vi "From Serial Form.vi"(6 "Serial Version":T1, 10 "Deserializer in":refnum<class "Deserializer.lvclass">, 11 "BrowerComponent in":refnum<class "BrowerComponent.lvclass">) -> (0 "error out":errorcluster, 2 "Deserializer out":refnum<class "Deserializer.lvclass">, 3 "BrowerComponent out":refnum<class "BrowerComponent.lvclass">)   [LabVIEW 2015, in "BrowerComponent.lvclass"]
uses:
  BrowerComponent.lvclass
  <vilib>/NI/AQ Character Lineator/Deserializer/Deserializer.lvclass
  <vilib>/NI/AQ Character Lineator/Serialization Common/Serial Version.ctl
  <vilib>/NI/AQ Character Lineator/Serializable/Remove String.vi
  <vilib>/NI/AQ Character Lineator/Serializable/Remove Int32.vi
  <vilib>/NI/AQ Character Lineator/Serializable Variant/Remove Variant.vi
  <vilib>/NI/AQ Character Lineator/Serializable/Serializable.lvclass
  <vilib>/NI/AQ Character Lineator/Serializable Variant/Serializable Variant.lvclass
  <vilib>/NI/AQ Character Lineator/Serialization Common/Serialization Common.lvlib
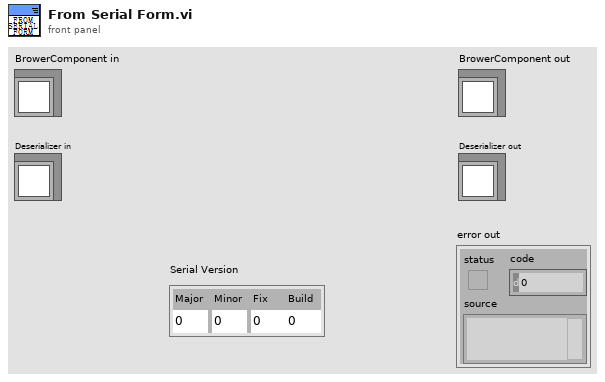
[diagram p1: front panel]
types:
  T1 = typedef "Serialization Common.lvlib/Serial Version.ctl" = cluster{"Major":u16, "Minor":u16, "Fix":u16, "Build":u16}
  T2 = typedef "BrowerComponent.lvclass/ObjectAttributes.ctl" = cluster{"ComponentID":string, "SymbolIndex":i32, "ComponentName":string, "PartsOfComponent_dict":variant}
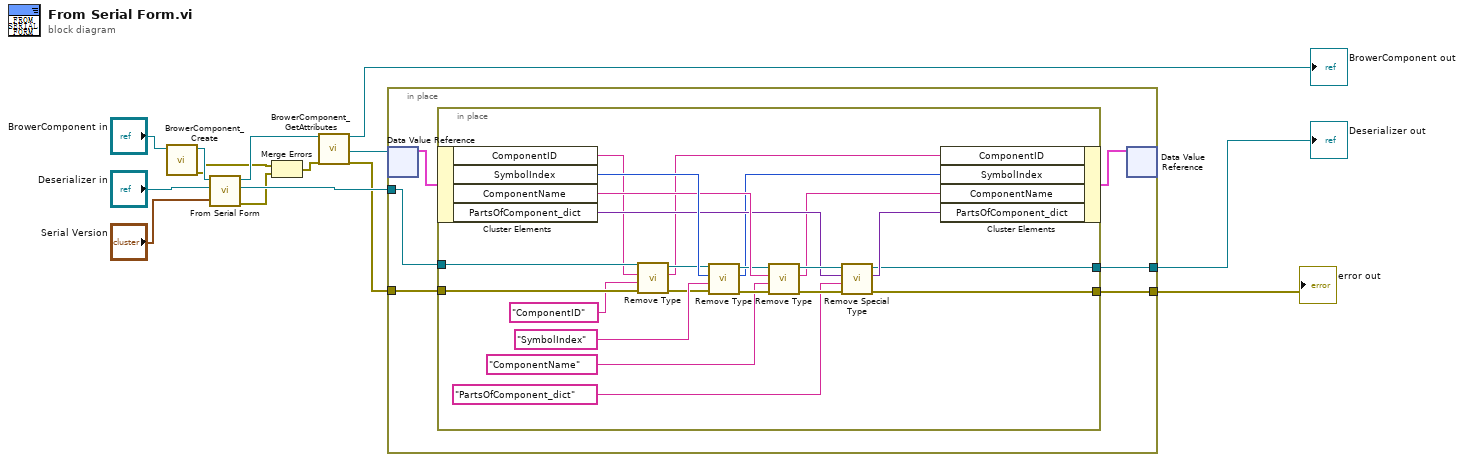
[diagram p0: block diagram]
diagram:
  n1 = call "BrowerComponent_Create.vi"("reference in"="BrowerComponent in") -> ("error out"=w3:errorcluster, "reference out"=w4:refnum<class "BrowerComponent.lvclass">)  [unwired: 9 in]
  n2 = call-parent "From Serial Form.vi"("Serial Version"="Serial Version", "Deserializer in"="Deserializer in", "Serializable in"=w4) -> ("error out"=w2:errorcluster, "Deserializer out"=w11:refnum<class "Deserializer.lvclass">, "Serializable out"=w6:refnum<class "BrowerComponent.lvclass">)  [unwired: 6 in]
  n3 = Merge Errors(w3, w2) -> (w1:errorcluster)
  n4 = call "BrowerComponent_GetAttributes.vi"("reference in"=w6, "error in (no error)"=w1) -> ("reference out"=→"BrowerComponent out":refnum<class "BrowerComponent.lvclass">, "DataRef"=w12:refnum<data-value>, "error out"=w7:errorcluster)  [unwired: 14 in, 1 out]
  n5 = in-place {
    in-place-border: w11 -> [w19]
    in-place-border: w7 -> [w18]
    in-place-border: [w16] -> w9
    in-place-border: [w15] -> w8
    n6 = in-place-dvr #1(w12) -> (w20:T2)  [unwired: 1 out]
    n7 = in-place {
      in-place-border: w19 -> [w42]
      in-place-border: w18 -> [w41]
      in-place-border: [w24] -> w16
      in-place-border: [w23] -> w15
      n8 = in-place-cluster #2(w20) -> ("ComponentID"=w22:string, "SymbolIndex"=w39:i32, "ComponentName"=w35:string, "PartsOfComponent_dict"=w29:variant)
      n9 = call-poly <vilib>:"Remove Type.vi"("error in (no error)"=w41, "Name"="ComponentID", "Default Value"=w22, "Deserializer in"=w42) -> ("error out"=w36:errorcluster, "String"=w21:string, "Deserializer out"=w38:refnum<class "Deserializer.lvclass">)  [unwired: 4 in, 1 out]
      n10 = call-poly <vilib>:"Remove Type.vi"("error in (no error)"=w36, "Name"="SymbolIndex", "Default Value"=w39, "Deserializer in"=w38) -> ("error out"=w33:errorcluster, "Numeric"=w25:i32, "Deserializer out"=w34:refnum<class "Deserializer.lvclass">)  [unwired: 4 in, 1 out]
      n11 = call-poly <vilib>:"Remove Type.vi"("error in (no error)"=w33, "Name"="ComponentName", "Default Value"=w35, "Deserializer in"=w34) -> ("error out"=w30:errorcluster, "String"=w26:string, "Deserializer out"=w31:refnum<class "Deserializer.lvclass">)  [unwired: 4 in, 1 out]
      n12 = call-poly <vilib>:"Remove Special Type.vi"("error in (no error)"=w30, "Name"="PartsOfComponent_dict", "Default Value"=w29, "Deserializer in"=w31) -> ("error out"=w23:errorcluster, "Variant"=w27:variant, "Deserializer out"=w24:refnum<class "Deserializer.lvclass">)  [unwired: 4 in, 1 out]
      n13 = in-place-cluster #2("ComponentID"=w21, "SymbolIndex"=w25, "ComponentName"=w26, "PartsOfComponent_dict"=w27) -> (w17:T2)
    }
    n14 = in-place-dvr #1(w17) -> ()  [unwired: 2 out]
  }
  "error out" <- w8
  "Deserializer out" <- w9
